vi "PCO_SetIntensifiedMCP.vi"(0 "ph":u64, 5 "wIntensifiedVoltage":u16, 7 "dwIntensifiedPhosphorDecay_us":u32, 11 "error in (no error)":errorcluster {"code" format="%x"}) -> (4 "ph out":u64, 6 "ErrorMessage":i32 format="%x", 15 "error out":errorcluster {"code" format="%x"})   [LabVIEW 2020, in "SDK.lvlib" / "SpecialCommandsDicam.lvlib"]
doc: "SC2_SDK_FUNC int WINAPI PCO_SetIntensifiedMCP(HANDLE ph, \n WORD wIntensifiedVoltage,\n WORD wFlags,\n WORD wReserved,\n DWORD dwIntensifiedPhosphorDecay_us,\n DWORD dwReserved1, DWORD dwReserved2);"
uses:
  SpecialCommandsDicam.lvlib
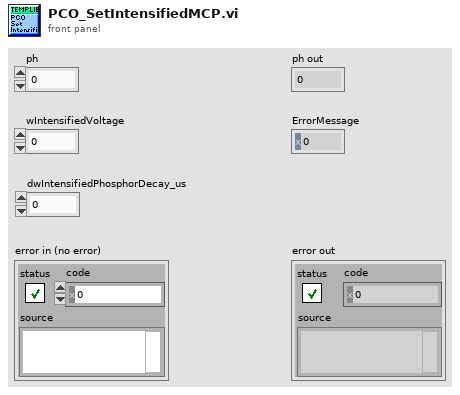
[diagram p1: front panel]
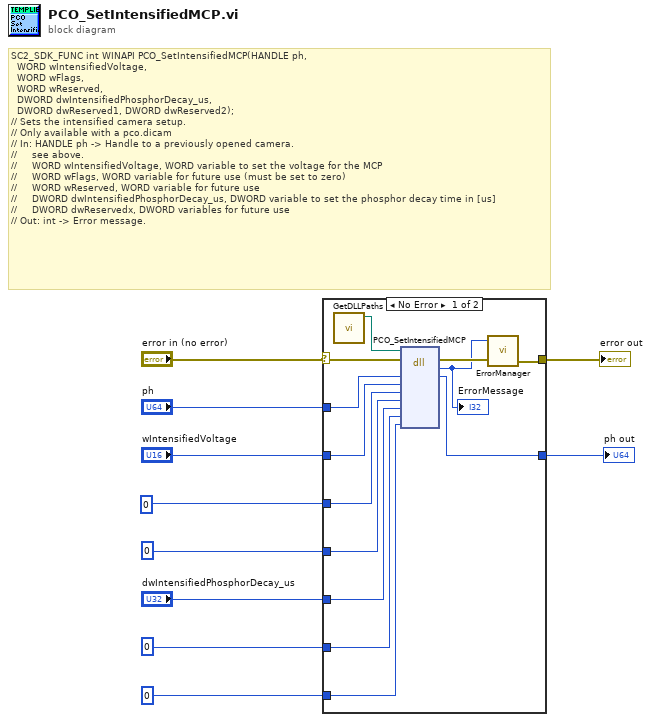
[diagram p0: block diagram]
diagram:
  # "SC2_SDK_FUNC int WINAPI PCO_SetIntensifiedMCP(HANDLE ph, \n  WORD wIntensifiedVoltage,\n  WORD wFlags,\n  WORD wReserved,\n  DWORD dwIntensifiedPhosphorDecay_us,\n  DWORD dwReserved1, DWORD dwReserved2);\n// Sets the intensified camera setup.\n// Only available with a pco.dicam\n// In: HANDLE ph -> Handle to a previously opened camera.\n//     see above.\n//     WORD wIntensifiedVoltage, WORD variable to set the voltage for the MCP\n//     WORD wFlags, WORD variable for future use (must be set to zero)\n//     WORD wReserved, WORD variable for future use \n//     DWORD dwIntensifiedPhosphorDecay_us, DWORD variable to set the phosphor decay time in [us]\n//     DWORD dwReservedx, DWORD variables for future use \n// Out: int -> Error message."
  n1 = case shown="No Error" "error in (no error)" {
    selector: "error in (no error)" -> [w15 w24]
    tunnel: "ph" -> [w23 w25]
    tunnel: [w22 w25] -> w9
    tunnel: "wIntensifiedVoltage" -> [w21 _]
    tunnel: u16 0 ("wFlags") -> [w20 _]
    tunnel: "dwIntensifiedPhosphorDecay_us" -> [w19 _]
    tunnel: [w14 w24] -> w6
    tunnel: u16 0 ("wReserved") -> [w18 _]
    tunnel: u32 0 ("dwReserved1") -> [w17 _]
    tunnel: u32 0 ("dwReserved2") -> [w16 _]
    frame No Error {
      n2 = call "GetDLLPaths.vi"() -> ("SC2_Cam_Path"=w11:path)  [unwired: 9 in, 2 out]
      n3 = dll-call lib="?" fn="PCO_SetIntensifiedMCP"(path in=w11, error in=w15, "ph"=w23, "wIntensifiedVoltage"=w21, "wFlags"=w20, "wReserved"=w18, "dwIntensifiedPhosphorDecay_us"=w19, "dwReserved1"=w17, "dwReserved2"=w16) -> (error out=w13:errorcluster, "return type"=w12:i32, "ph"=w22:u64)  [unwired: 7 in, 1 out]
      "ErrorMessage" <- w12
      n4 = call "ErrorManager.vi"("error in (no error)"=w13, "error code"=w12) -> ("error out"=w14:errorcluster)  [unwired: 3 in]
    }
    frame Error {
    }
  }
  "ph out" <- w9
  "error out" <- w6
